vi "Apply breakpoints and rates.vi"(8 "error in (no error)":errorcluster, 10 "Ramp rate (A/sec)":dbl format="%#_13g", 11 "PS Driver in":refnum<class "PS Driver.lvclass">) -> (0 "error out":errorcluster, 1 "Rates (A/sec)":dbl[](array[numeric]), 2 "Breakpoints (A)":dbl[](array[numeric]), 3 "PS Driver out":refnum<class "PS Driver.lvclass">)   [LabVIEW 2025, in "PS Driver.lvlib" / "PS Driver.lvclass"]
doc: "Author: Scott Hannahs <sth@magnet.fsu.edu>\n\nThis software is licensed for use under the “MIT License\"\nCopyright (c) 2025 Scott Hannahs, sth@sth@magnet.sthnet.net\n\nPermission is hereby granted, free of charge, to any person obtaining a copy of this software and associated documentation files (the \"Software\"), to deal in the Software without restriction, including without limitation the rights to use, copy, modify, merge, publish, distribute, sublicense, and/or sell copies of the Software, and to permit persons to whom the Software is furnished to do so, subject to the following conditions: The above copyright notice and this permission notice shall be included in all copies or substantial portions of the Software.\n\nTHE SOFTWARE IS PROVIDED \"AS IS\", WITHOUT WARRANTY OF ANY KIND, EXPRESS OR IMPLIED, INCLUDING BUT NOT LIMITED TO THE WARRANTIES OF MERCHANTABILITY, FITNESS FOR A PARTICULAR PURPOSE AND NONINFRINGEMENT. IN NO EVENT SHALL THE AUTHORS OR COPYRIGHT HOLDERS BE LIABLE FOR ANY CLAIM, DAMAGES OR OTHER LIABILITY, WHETHER IN AN ACTION OF CONTRACT, TORT OR OTHERWISE, ARISING FROM, OUT OF OR IN CONNECTION WITH THE SOFTWARE OR THE USE OR OTHER DEALINGS IN THE SOFTWARE."
uses:
  PS Driver.lvclass
  PS Driver.lvclass/PS Driver.ctl
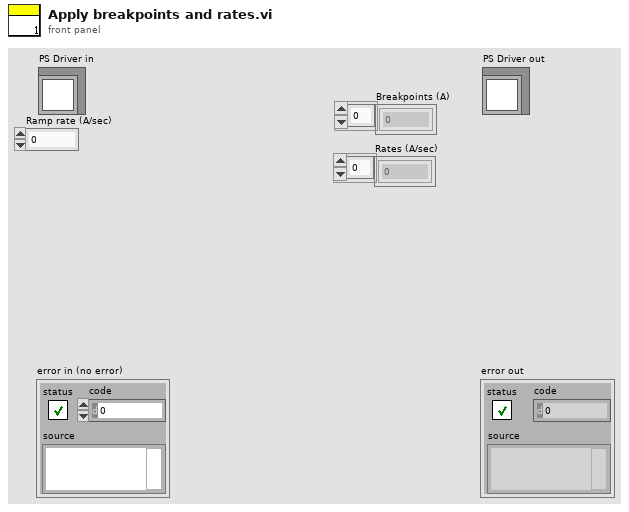
[diagram p1: front panel]
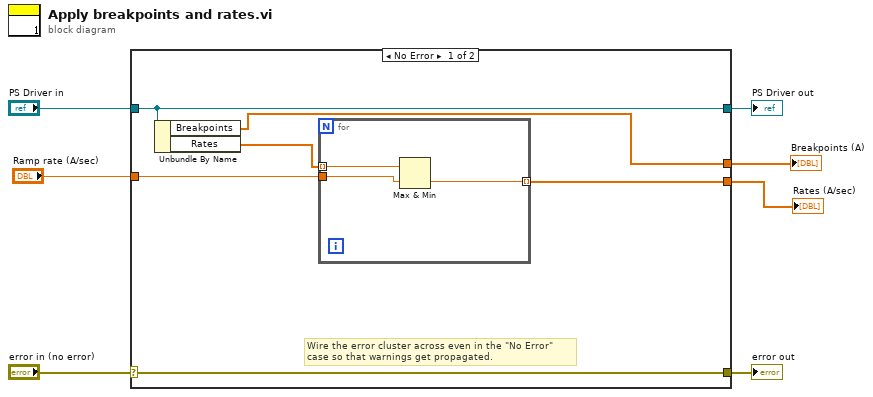
[diagram p0: block diagram]
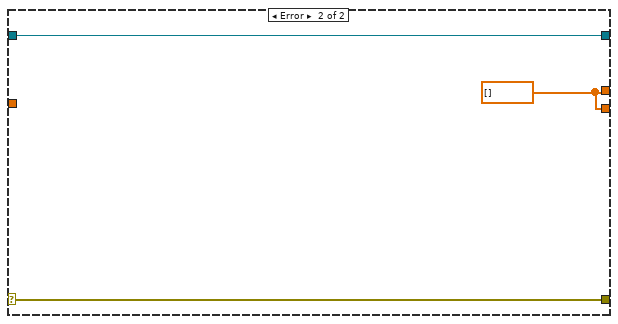
[diagram p2: hidden frame]
diagram:
  n1 = case shown="No Error" "error in (no error)" {
    selector: "error in (no error)" -> [w13 w19]
    tunnel: [w13 w19] -> w6
    tunnel: [w12 w18] -> w4
    tunnel: "PS Driver in" -> [w12 w18]
    tunnel: "Ramp rate (A/sec)" -> [w10 _]
    tunnel: [w9 w17] -> w2
    tunnel: [w8 w17] -> w1
    frame No Error {
      # "Wire the error cluster across even in the \"No Error\"\ncase so that warnings get propagated."
      n2 = Unbundle By Name(w12) -> ("Breakpoints"=w8:dbl[], "Rates"=w11:dbl[])
      n3 = for {
        tunnel: w11 -> [w16] mode=indexing
        tunnel: w10 -> [w15]
        tunnel: [w14] -> w9 mode=indexing
        n4 = Max & Min(x=w16, y=w15) -> (min(x,y)=w14:dbl)  [unwired: 1 out]
      }
    }
    frame Error {
      w17 = dbl[] []
    }
  }
  "error out" <- w6
  "PS Driver out" <- w4
  "Rates (A/sec)" <- w2
  "Breakpoints (A)" <- w1
